vi "Clear Snapshot.vi"(6 "IPath Getter.lvclass":refnum<class "IPath Getter.lvclass">, 8 "error in":errorcluster, 11 "VI Reference in":refnum<vi>) -> (0 "error out":errorcluster, 3 "VI Reference out":refnum<vi>)   [LabVIEW 2020, in "Public API.lvlib"]
doc: "Clear the <b>Debug Snapshot</b> of the active VI from the Cache File."
uses:
  Public API.lvlib
  IPath Getter/IPath Getter.lvclass
  Type Definitions/Debug Snapshot Array--cluster.ctl
  Type Definitions/Debug Snapshot--cluster.ctl
  Type Definitions/Breakpoint--cluster.ctl
  <vilib>/Utility/miscctls.llb/LVBreakpointStatusEnum.ctl
  Type Definitions/Class Name--enum.ctl
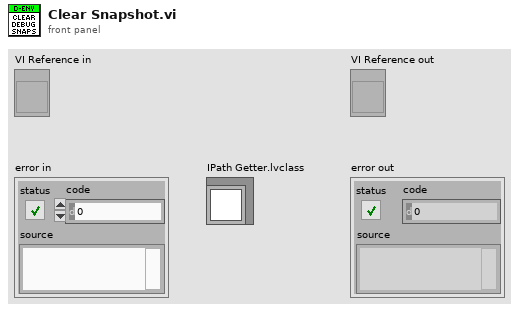
[diagram p1: front panel]
types:
  T1 = typedef "Debug Snapshot Array--cluster.ctl" = cluster{"Debug Snapshots":T2[]}
  T2 = typedef "Debug Snapshot--cluster.ctl" = cluster{"VI Name":string, "Breakpoints":T3[], "Probes":i32[]}
  T3 = typedef "Breakpoint--cluster.ctl" = cluster{"UID":i32, "BP Status":T4, "Class Name":T5}
  T4 = typedef "LVBreakpointStatusEnum.ctl" = enum8{"Cleared Break", "Enabled Break", "Disabled Break"}
  T5 = typedef "Class Name--enum.ctl" = enum16{"Node", "Wire"}
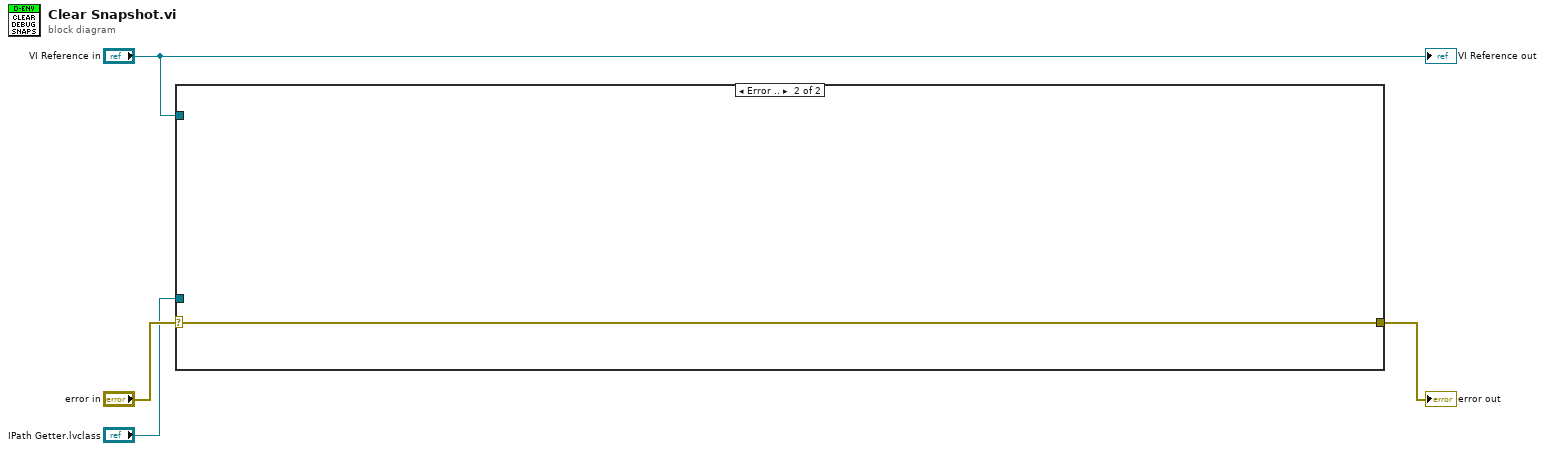
[diagram p0: block diagram]
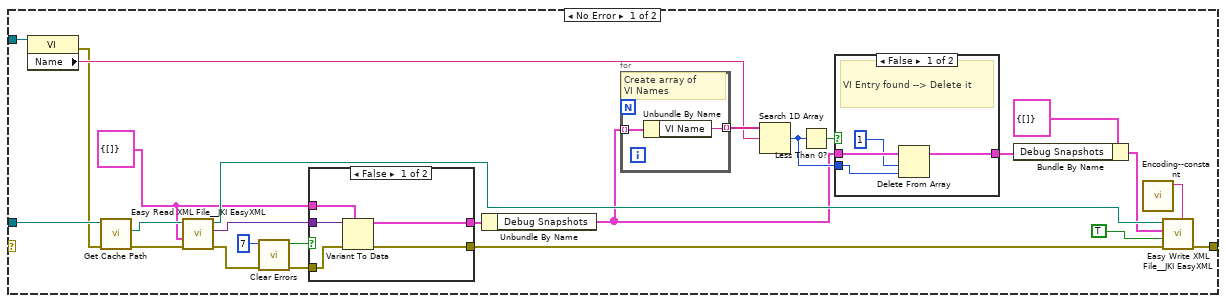
[diagram p2: hidden frame]
diagram:
  n1 = case shown="Error .." "error in" {
    selector: "error in" -> [_ w43]
    tunnel: [w27 w43] -> w3
    tunnel: "VI Reference in" -> [w29 _]
    tunnel: "IPath Getter.lvclass" -> [w14 _]
    frame No Error {
      w10 = T1 {"Debug Snapshots"=[]} ("Debug Snapshot Array")
      n2 = property class="VI"(reference=w29) -> (error out=w12:errorcluster, "Name"=w22:string)  [unwired: 1 in, 1 out]
      n3 = call-dynamic "Get Cache Path.vi"("error in (no error)"=w12, "IPath Getter in"=w14) -> ("error out"=w11:errorcluster, "Path"=w13:path)  [unwired: 8 in]
      n4 = call <vilib>:"Easy Read XML File__JKI EasyXML.vi"("error in (no error)"=w11, "LabVIEW Data (Type)"=w10, "XML File Path"=w13) -> ("error out"=w17:errorcluster, "LabVIEW Data"=w26:variant, "XML File Path (duplicate)"=w20:path)  [unwired: 6 in]
      n5 = call <vilib>:"Clear Errors.vi"("error in (no error)"=w17, "specific error code to clear (0: all)"=7) -> ("error out"=w16:errorcluster, "specific error cleared?"=w15:bool)  [unwired: 4 in]
      n6 = case shown="False" w15 {
        tunnel: w26 -> [w34 _]
        tunnel: w10 -> [w33 _]
        tunnel: [w32 _] -> w9
        tunnel: [w31 w35] -> w21
        tunnel: w16 -> [w30 w35]
        frame False {
          n7 = Variant To Data(error in=w30, type=w33, Variant=w34) -> (data=w32:T1, error out=w31:errorcluster)
        }
        frame True {
        }
      }
      n8 = Unbundle By Name(w9) -> ("Debug Snapshots"=w8:T2[])
      n9 = for {
        tunnel: w8 -> [w42] mode=indexing
        tunnel: [w41] -> w25 mode=indexing
        # "Create array of\nVI Names"
        n10 = Unbundle By Name(w42) -> ("VI Name"=w41:string)
      }
      n11 = Search 1D Array(1D array=w25, element=w22) -> (index of element=w23:i32)  [unwired: 1 in]
      n12 = Less Than 0?(x=w23) -> (x < 0?=w24:bool)
      n13 = case shown="False" w24 {
        tunnel: w8 -> [w39 w40]
        tunnel: [w38 w40] -> w6
        tunnel: w23 -> [w37 _]
        frame False {
          # "VI Entry found --> Delete it"
          n14 = Delete From Array(array=w39, length=1, index=w37) -> (array with subset deleted=w38:T2[])  [unwired: 1 out]
        }
        frame True {
          # "Entry does not exist."
        }
      }
      n15 = Bundle By Name(cluster=T1 {"Debug Snapshots"=[]} ("Debug Snapshot Array"), "Debug Snapshots"=w6) -> (w5:T1)
      n16 = call "Encoding--constant.vi"() -> ("Encoding (none)"=w28:string)  [unwired: 11 in]
      n17 = call <vilib>:"Easy Write XML File__JKI EasyXML.vi"("Encoding (none)"=w28, "error in (no error)"=w21, "Overwrite File? (false)"=TRUE, "LabVIEW Data"=w5, "XML File Path"=w20) -> ("error out"=w27:errorcluster)  [unwired: 5 in, 1 out]
    }
    frame Error {
    }
  }
  "error out" <- w3
  "VI Reference out" <- "VI Reference in"
